vi "calculatePitch.vi"(9 "az":dbl, 10 "ay":dbl, 11 "ax":dbl) -> (3 "pitch":dbl)   [LabVIEW 2015]
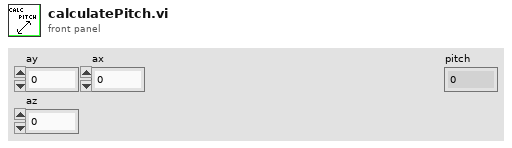
[diagram p1: front panel]
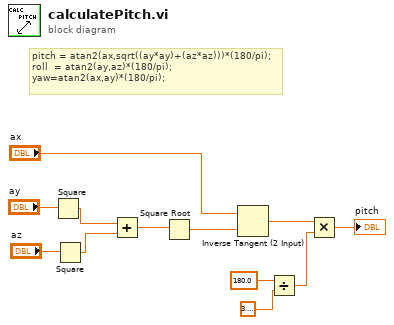
[diagram p0: block diagram]
diagram:
  # "pitch = atan2(ax,sqrt((ay*ay)+(az*az)))*(180/pi);\nroll  = atan2(ay,az)*(180/pi);\nyaw=atan2(ax,ay)*(180/pi);"
  n1 = Square(x="ay") -> (x^2=w9:dbl)
  n2 = Square(x="az") -> (x^2=w10:dbl)
  n3 = Add(x=w9, y=w10) -> (x+y=w8:dbl)
  n4 = Square Root(x=w8) -> (sqrt(x)=w6:dbl)
  n5 = Inverse Tangent (2 Input)(1:w6, 2:"ax") -> (0:w5:dbl)
  n6 = Divide(x=180.0, y=3.141592653589793) -> (x/y=w2:dbl)
  n7 = Multiply(x=w5, y=w2) -> (x*y=→"pitch":dbl)
